vi "Set Pin Infos.vi"(0 "Display State In":T3, 7 "Pin Info Array":T1, 9 "Container State":T4, 11 "error in (no error)":errorcluster) -> (4 "Display State Out":T3, 15 "error out":errorcluster)   [LabVIEW 2021, in "roboRIO SPI.xctl"]
uses:
  <vilib>/myRIO/Common/Instrument Driver Framework/Utilities/xctls/roboRIO SPI/roboRIO SPI.xctl
  <vilib>/_xctls/Container State.ctl
  <vilib>/myRIO/Common/Instrument Driver Framework/Utilities/xctls/roboRIO SPI/State.ctl
  <vilib>/myRIO/Common/Instrument Driver Framework/Utilities/xctls/utilities/typedefs/myRIOXC Pin Info Array.ctl
  <vilib>/myRIO/Common/Instrument Driver Framework/Utilities/xctls/utilities/typedefs/myRIOXC Pin Info.ctl
  <vilib>/myRIO/Common/Instrument Driver Framework/Utilities/xctls/utilities/vis/myRIOXC Set Pin Info.vi
  <vilib>/_xctls/XControlSupport.lvlib
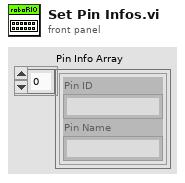
[diagram p1: front panel]
types:
  T1 = typedef "myRIOXC Pin Info Array.ctl" = T2[]
  T2 = typedef "myRIOXC Pin Info.ctl" = cluster{"Pin ID":string, "Pin Name":string}
  T3 = typedef "roboRIO SPI.xctl/State.ctl" = cluster{"Pin Disabled?":enum8{"Enabled", "Disabled", "Disabled and Grayed Out"}[], "Pin Name":string[]}
  T4 = typedef "XControlSupport.lvlib/Container State.ctl" = cluster{"Indicator?":bool, "Run Mode?":bool, " Refnum":refnum<vi>}
  T5 = typedef "myRIOXC Display State.ctl" = cluster{"Pin Disabled?":enum8{"Enabled", "Disabled", "Disabled and Grayed Out"}[], "Pin Name":string[]}
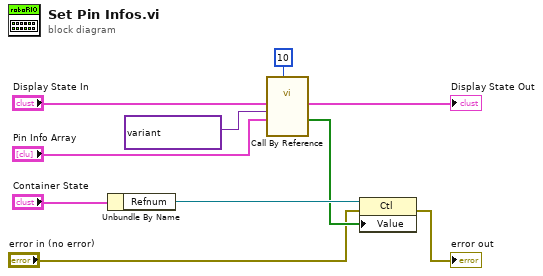
[diagram p0: block diagram]
diagram:
  n1 = Unbundle By Name("Container State") -> ("Refnum"=w6:refnum<vi>)
  n2 = call-by-ref "?"("Size"=10, "Pin Name Array"="Pin Info Array", "Pin ID Map"=variant("Pin 1"=variant(i32 0), "Pin 10"=variant(i32 9), "Pin 2"=variant(i32 1), "Pin 3"=variant(i32 2), "Pin 4"=variant(i32 3), "Pin 5"=variant(i32 4), "Pin 6"=variant(i32 5), "Pin 7"=variant(i32 6), "Pin 8"=variant(i32 7), "Pin 9"=variant(i32 8)) ("variant"), "Display State In in"="Display State In") -> ("Data"=w5:bool[], "Display State In out"=→"Display State Out":T5)  [unwired: 8 in, 2 out]
  n3 = property class="Ctl"(reference=w6, error in="error in (no error)", "Value"=w5) -> (error out=→"error out":errorcluster)  [unwired: 1 out]
